vi "VariablesLocales_conGlobalesFuncionales.vi"() -> ()   [LabVIEW 2020]
panel:
  out "Waveform Chart 2":dbl(graph)
  out "Waveform Chart":dbl(graph)
  in  "Boton de paro de ambas":bool
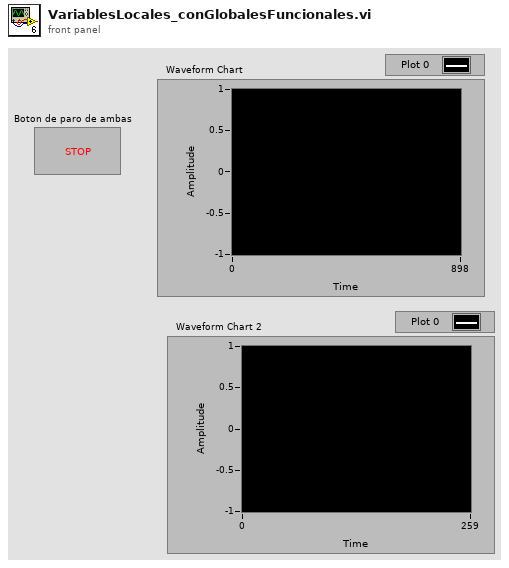
[diagram p1: front panel]
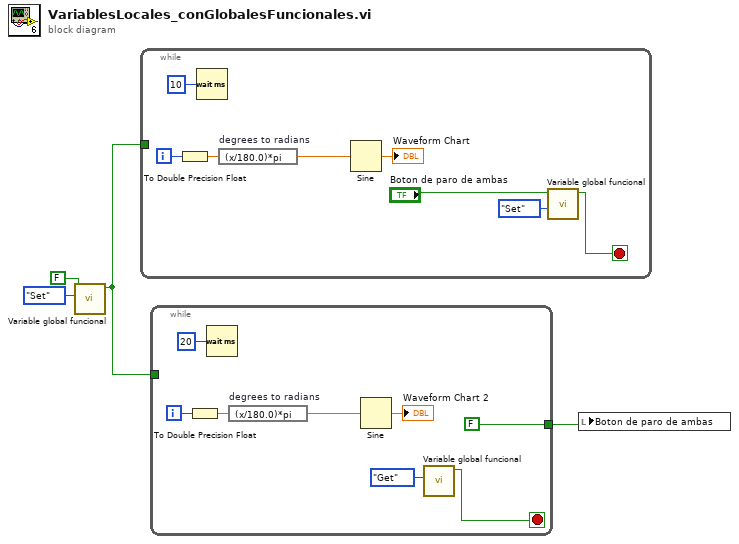
[diagram p0: block diagram]
diagram:
  n1 = call "Variable global funcional.vi"("Action"=enum16{"Get", "Set"}."Set", "New value"=FALSE) -> ("Output value"=w1:bool)  [unwired: 9 in]
  n2 = while {
    tunnel: w1 -> [_]
    i -> [w10]
    stop <- w5 stop-if-true
    n3 = To Double Precision Float(number=w10) -> (double precision float=w9:dbl)
    n4 = Wait (ms)(milliseconds to wait=u32 10) -> ()  [unwired: 1 out]
    n5 = expression code="(x/180.0)*pi" "degrees to radians"(w9) -> (w11:dbl)
    n6 = Sine(x=w11) -> (sin(x)=→"Waveform Chart":dbl)
    n7 = call "Variable global funcional.vi"("Action"=enum16{"Get", "Set"}."Set", "New value"="Boton de paro de ambas") -> ("Output value"=w5:bool)  [unwired: 9 in]
  }
  n8 = while {
    tunnel: [FALSE] -> w4
    tunnel: w1 -> [_]
    i -> [w18]
    stop <- w13 stop-if-true
    n9 = To Double Precision Float(number=w18) -> (double precision float=w17:dbl)
    n10 = Wait (ms)(milliseconds to wait=u32 20) -> ()  [unwired: 1 out]
    n11 = expression code="(x/180.0)*pi" "degrees to radians"(w17) -> (w19:dbl)
    n12 = Sine(x=w19) -> (sin(x)=→"Waveform Chart 2":dbl)
    n13 = call "Variable global funcional.vi"("Action"=enum16{"Get", "Set"}."Get") -> ("Output value"=w13:bool)  [unwired: 10 in]
  }
  n14 = local write "Boton de paro de ambas"(w4) -> ()
